vi "AUTOFLIM_Draw_emitters.vi"(6 "Y Scan Range":dbl, 8 "error in (no error)":errorcluster, 9 "X Scan Range":dbl, 10 "Mesh":dbl, 11 "cent":i32[][](array[numeric])) -> (0 "error out":errorcluster, 3 "Plot Images:Front":picture)   [LabVIEW 2023]
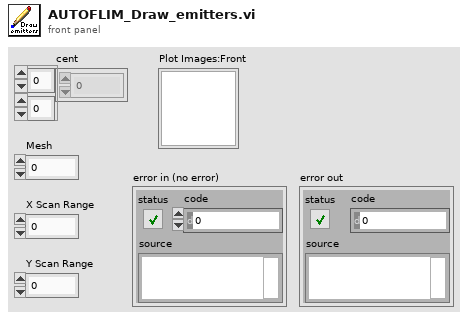
[diagram p1: front panel]
types:
  T1 = cluster{"Font Name:":string, "Size":i16, "Strikeout?":bool, "Italic?":bool, "Underline?":bool, "Outline?":bool, "Shadow?":bool, "Bold?":bool}
  T2 = enum16{"None", "Stacked", "Clockwise", "Counterclockwise"}
  T3 = cluster{"Width":u16, "Style":enum32{"Solid", "Dash", "Dot", "DashDot", "DashDotDot"}}
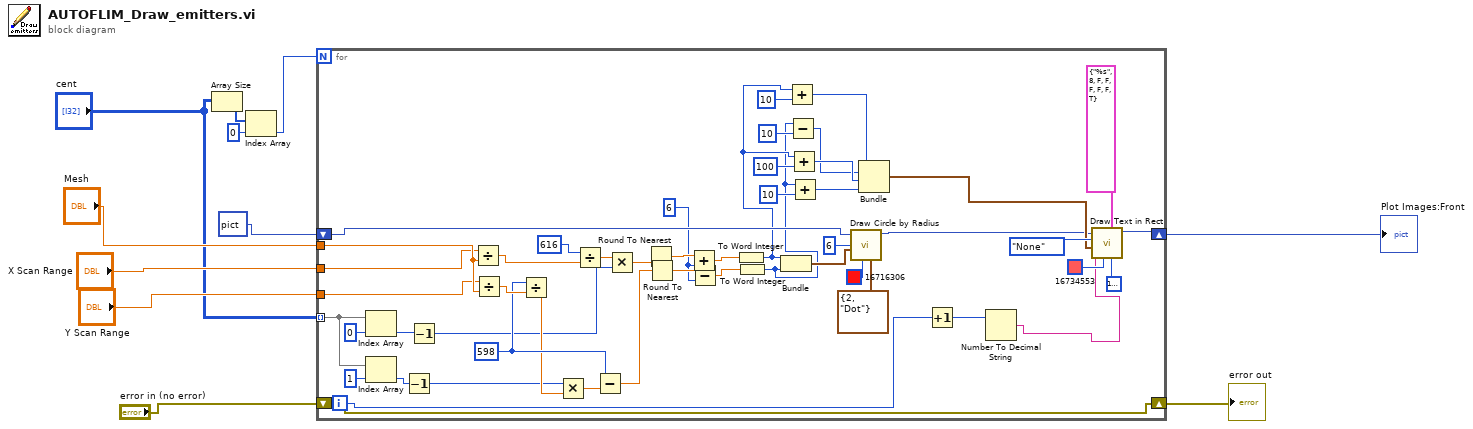
[diagram p0: block diagram]
diagram:
  n1 = Array Size(array="cent") -> (size(s)=w5:i32[])
  n2 = Index Array(array=w5, index=0) -> (element=w7:i32)
  n3 = for {
    N: w7 -> [_]
    tunnel: "cent" -> [w60] mode=indexing
    shift-right: [w24] -> w3
    shift-left: picture data[5B] ("Plot Images:Front") -> [w58]
    tunnel: "Mesh" -> [w20]
    tunnel: "X Scan Range" -> [w19]
    tunnel: "Y Scan Range" -> [w18]
    shift-right: [w17] -> w1
    shift-left: "error in (no error)" -> [w17]
    i -> [w22]
    w12 = 6
    w46 = i16 598 ("x")
    n4 = Index Array(array=w60, index=0) -> (element=w28:i32)
    n5 = Index Array(array=w60, index=1) -> (element=w29:i32)
    n6 = Decrement(x=w29) -> (x-1=w26:i32)
    n7 = Decrement(x=w28) -> (x-1=w27:i32)
    n8 = Divide(x=w19, y=w20) -> (x/y=w49:dbl)
    n9 = Divide(x=w18, y=w20) -> (x/y=w47:dbl)
    n10 = Divide(x=w46, y=w47) -> (x/y=w45:dbl)
    n11 = Multiply(x=w26, y=w45) -> (x*y=w53:dbl)
    n12 = Divide(x=616, y=w49) -> (x/y=w48:dbl)
    n13 = Subtract(x=w46, y=w53) -> (x-y=w52:dbl)
    n14 = Multiply(x=w48, y=w27) -> (x*y=w51:dbl)
    n15 = Round To Nearest(number=w51) -> (nearest integer value=w14:dbl)
    n16 = Round To Nearest(number=w52) -> (nearest integer value=w13:dbl)
    n17 = Add(x=w14, y=w12) -> (x+y=w16:dbl)
    n18 = Subtract(x=w13, y=w12) -> (x-y=w15:dbl)
    n19 = To Word Integer(number=w16) -> (16bit integer=w37:i16)
    n20 = To Word Integer(number=w15) -> (16bit integer=w36:i16)
    n21 = Bundle(w37, w36) -> (w54:cluster{i16, i16})  [unwired: 1 in]
    n22 = Add(x=w37, y=i16 10) -> (x+y=w32:i16)
    n23 = Subtract(x=w36, y=i16 10) -> (x-y=w33:i16)
    n24 = Add(x=w37, y=i16 100) -> (x+y=w34:i16)
    n25 = Add(x=w36, y=i16 10) -> (x+y=w35:i16)
    n26 = call <vilib>:"Draw Circle by Radius.vi"("pen"=T3 {"Width"=2, "Style"=enum."Dot"}, "color(black)"=u32 16716306, "pixel center"=w54, "radius"=i16 6, "picture"=w58) -> ("new picture"=w25:picture)  [unwired: 6 in]
    n27 = Bundle(w32, w33, w34, w35) -> (w42:cluster{i16, i16, i16, i16})  [unwired: 1 in]
    n28 = Increment(x=w22) -> (x+1=w21:i32)
    n29 = Number To Decimal String(number=w21) -> (decimal integer string=w23:string)  [unwired: 1 in]
    n30 = call <vilib>:"Draw Text in Rect.vi"("BG color(transparent)"=u32 16777216, "[user-specified font]"=T1 {"Font Name:"="%s", "Size"=8, "Strikeout?"=FALSE, "Italic?"=FALSE, "Underline?"=FALSE, "Outline?"=FALSE, "Shadow?"=FALSE, "Bold?"=TRUE}, "text color(black)"=u32 16734553, "text"=w23, "rect"=w42, "text orientation"=T2."None", "picture"=w25) -> ("new picture"=w24:picture)  [unwired: 4 in]
  }
  "Plot Images:Front" <- w3
  "error out" <- w1
